vi "FromRepo.vi"(8 "error in":errorcluster, 9 "from repo cluster":T2, 10 "repository in":refnum<class "NISE_CEF_Repository.lvclass">, 11 "node in":refnum<class "RunTimeObjectsSection.lvclass">) -> (0 "error out":errorcluster, 2 "repository out":refnum<class "NISE_CEF_Repository.lvclass">, 3 "node":T1)   [LabVIEW 2015, in "RunTimeObjectsSection.lvclass"]
doc: "Grabs information from the Repo and stores it in the nodes."
uses:
  RunTimeObjectsSection.lvclass
  <vilib>/NI/Configuration Framework/Repository/NISE_CEF_Repository.lvclass
  <vilib>/NI/Configuration Framework/Node/FromRepoCluster.ctl
  <vilib>/NI/Configuration Framework/Node/NodeRef.ctl
  <vilib>/NI/Configuration Framework/Node/NISE_CEF_Node.lvclass
  CustomDeviceRepo/CustomDeviceRepo.lvclass
  Controls/RunTimeObjectTypes.ctl
  Controls/RunTimeObjectsVariantCluster.ctl
  CustomDeviceRepo/CustomDeviceRepo.lvclass/CustomDeviceRepo.ctl
  RunTimeObjectsSection.lvclass/RunTimeObjectsSection.ctl
  CustomDeviceRepo/Read All Pages Properties.vi
  Write Section Name.vi
  Write RunTimeObjectType.vi
  Configuration Tool.lvlib
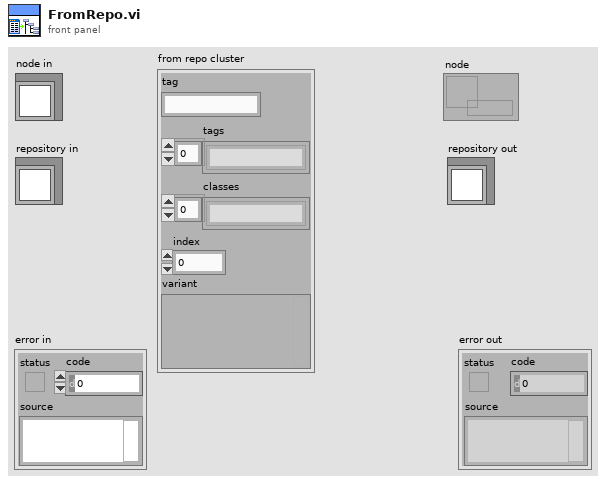
[diagram p1: front panel]
types:
  T1 = typedef "NISE_CEF_Node.lvclass/NodeRef.ctl" = refnum<data-value>
  T2 = typedef "NISE_CEF_Node.lvclass/FromRepoCluster.ctl" = cluster{"tag":string, "tags":string[], "classes":string[], "index":i32, "variant":variant}
  T3 = typedef "Configuration Tool.lvlib/RunTimeObjectsVariantCluster.ctl" = cluster{"Page Index":i32, "ActionVI Indexes":i32[]}
  T4 = typedef "Configuration Tool.lvlib/RunTimeObjectTypes.ctl" = enum16{"ActionVIs", "ButtonList", "RunTimeMenu"}
  T5 = typedef "Page Properties.ctl" = cluster{"Name":string, "Disallow Renaming":bool, "Delete Protection":bool, "Exlcude from Alphabetical order":bool, "Allow Multi-Selection":bool, "GUID":string, "Parent GUIDs":string[], "Glyph":T6, "Inactive Glyph":T6, "Broken Glyph":T6, "Item to Launch":T6, "Additional Information":string, "Copy":enum16{"copy", "disabled"}, "Paste":enum16{"Create", "CreatIfNotExists_GUID", "CreatIfNotExists_Name", "Replace", "Dialog"}, "Help":T7}
  T6 = typedef "Path Cluster.ctl" = cluster{"Path":path, "Path Type":enum16{"Absolute", "To Base", "To Common Doc Dir", "To Application Data Dir"}}
  T7 = typedef "help.ctl" = cluster{"Item to Launch":T6, "Section":string, "File Type":enum16{"chm", "other"}}
  T8 = typedef "ActionVIs Properties.ctl" = cluster{"Action VI On Delete":T6, "Action VI On Load":T6, "Action VI On Paste":T6, "Action VI On Target Type Change":T6, "Action VI On Delete Request":T6, "Action VI On Compile":T6, "Action VI On System Shutdown":T6, "Action VI On Save":T6, "Action VI On Download":T6}
  T9 = typedef "ButtonLists Properties.ctl" = cluster{"ID":string, "Glyph":T6, "Button Type":T10, "Referenced GUID":string, "Button Text":string, "Caption":string, "Tip Strip":string, "Documentation":string, "Dependency":T11}
  T10 = typedef "Button Type.ctl" = enum16{"Action", "Dialog", "Page", "Notification", "Separator"}
  T11 = typedef "Dependency three item small.ctl" = cluster{"File Path Control":path, "Path Type":enum16{"Absolute", "To Base", "To Common Doc Dir", "To Application Data Dir"}, "Behavior":enum16{"Static", "Dynamic"}}
  T12 = typedef "RunTimeMenus Properties.ctl" = cluster{"GUID":string, "Execution":T13, "MinNrOfChilds":u32, "Name":string, "Item to Launch":T6, "Dependency":T11, "Custom Population":T6, "Menu Item Type":enum16{"Action", "VI", "Separator", "Custom"}, "Behavior":enum16{"Nothing", "Open Front Panel"}, "Position":enum16{"Centered", "Mouse Pointer"}}
  T13 = typedef "Execution Types.ctl" = enum16{"silent", "modal", "floating", "default"}
  T14 = cluster{"General Page Properties":T5, "ActionVIs Properties":T8, "Button List Properties":T9[], "RunTime Menus Properties":T12[]}[]
  T15 = cluster{"General Page Properties":T5, "ActionVIs Properties":T8, "Button List Properties":T9[], "RunTime Menus Properties":T12[]}
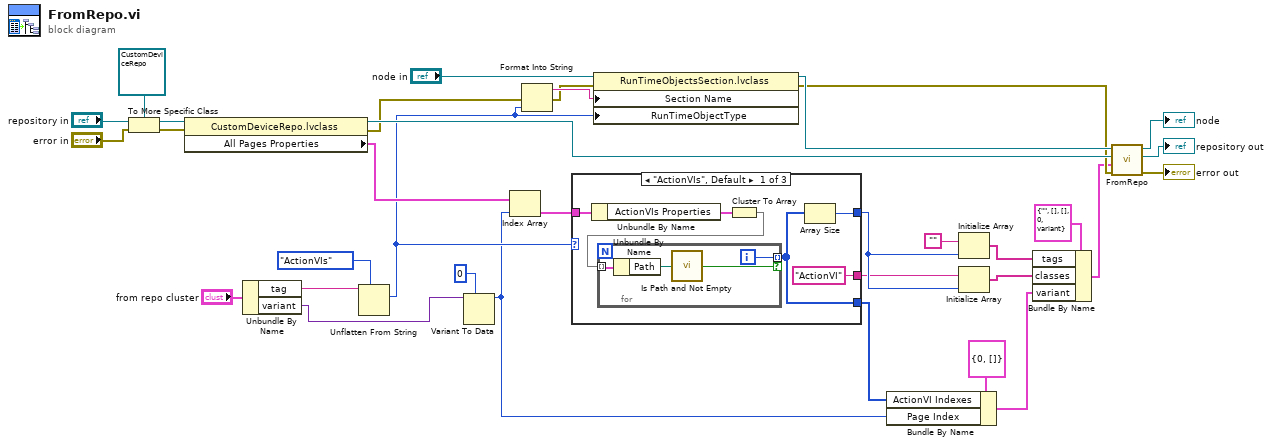
[diagram p0: block diagram]
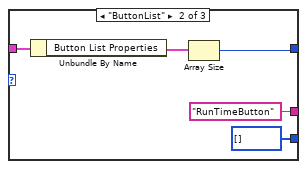
[diagram p2: hidden frame]
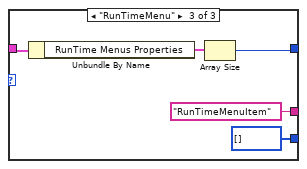
[diagram p3: hidden frame]
diagram:
  n1 = To More Specific Class(target class=refnum<class "CustomDeviceRepo.lvclass"> refnum ("CustomDeviceRepo.lvclass"), reference="repository in", error in="error in") -> (specific class reference=w30:refnum<class "CustomDeviceRepo.lvclass">, error out=w31:errorcluster)
  n2 = property class="CustomDeviceRepo.lvclass"(reference=w30, error in=w31) -> (reference out=w20:refnum<class "CustomDeviceRepo.lvclass">, error out=w19:errorcluster, "All Pages Properties"=w14:T14)
  n3 = Unbundle By Name("from repo cluster") -> ("tag"=w24:string, "variant"=w6:variant)
  n4 = Unflatten From String(type=RunTimeObjectTypes."ActionVIs" ("RunTimeObjectType"), binary string=w24) -> (value=w13:T4)  [unwired: 3 in, 2 out]
  n5 = Variant To Data(type=0, Variant=w6) -> (data=w4:i32)  [unwired: 1 in, 1 out]
  n6 = Index Array(array=w14, index=w4) -> (element=w1:T15)
  n7 = Format Into String(error in=w19, w13) -> (resulting string=w22:string, error out=w18:errorcluster)  [unwired: 2 in]
  n8 = case shown="\"ActionVIs\", Default" w13 {
    tunnel: w1 -> [w40 w49 w53]
    tunnel: [w36 w47 w51] -> w12
    tunnel: ["ActionVI" "RunTimeButton" "RunTimeMenuItem"] -> w8
    tunnel: [w35 i32[] [] ("ActionVI Indexes") i32[] [] ("ActionVI Indexes")] -> w3
    frame "ActionVIs", Default {
      n9 = Unbundle By Name(w40) -> ("ActionVIs Properties"=w39:T8)
      n10 = Cluster To Array(cluster=w39) -> (array=w37:T6[])
      n11 = for {
        tunnel: w37 -> [w44] mode=indexing
        tunnel: [w43] -> w35 mode=indexing if=w41
        i -> [w43]
        n12 = Unbundle By Name(w44) -> ("Path"=w42:path)
        n13 = call <vilib>:"Is Path and Not Empty.vi"("path"=w42) -> ("Is Path and Not Empty?"=w41:bool)  [unwired: 4 in]
      }
      n14 = Array Size(array=w35) -> (size(s)=w36:i32)
    }
    frame "ButtonList" {
      n15 = Unbundle By Name(w49) -> ("Button List Properties"=w48:T9[])
      n16 = Array Size(array=w48) -> (size(s)=w47:i32)
    }
    frame "RunTimeMenu" {
      n17 = Unbundle By Name(w53) -> ("RunTime Menus Properties"=w52:T12[])
      n18 = Array Size(array=w52) -> (size(s)=w51:i32)
    }
  }
  n19 = property class="RunTimeObjectsSection.lvclass"(reference="node in", error in=w18, "Section Name"=w22, "RunTimeObjectType"=w13) -> (reference out=w21:refnum<class "RunTimeObjectsSection.lvclass">, error out=w17:errorcluster)
  n20 = Bundle By Name(cluster=T3 {"Page Index"=0, "ActionVI Indexes"=[]}, "ActionVI Indexes"=w3, "Page Index"=w4) -> (w2:T3)
  n21 = Initialize Array("", w12) -> (w10:string[])
  n22 = Initialize Array(w8, w12) -> (w9:string[])
  n23 = Bundle By Name(cluster=T2 {"tag"="", "tags"=[], "classes"=[], "index"=0, "variant"=variant} ("from repo cluster"), "tags"=w10, "classes"=w9, "variant"=w2) -> (w7:T2)
  n24 = call-parent "FromRepo.vi"("error in"=w17, "from repo cluster"=w7, "repository in"=w20, "node in"=w21) -> ("error out"=→"error out":errorcluster, "repository out"=→"repository out":refnum<class "NISE_CEF_Repository.lvclass">, "node"=→"node":T1)  [unwired: 5 in]
